vi "CANopen add SDO from EDS.vi"(10 "SDO Parameters in":T4[](array[typedef]) {"Block Data" format="%.0x"}, 11 "Cluster":T2 {"ObjectType" items=[""=10, "NULL"=0, "DOMAIN"=2, "DEFTYPE"=5, "DEFSTRUCT"=6, "VAR"=7, "ARRAY"=8, "RECORD"=9]; "DataType" items=[""=0, "BOOLEAN"=1, "INTEGER8"=2, "INTEGER16"=3, "INTEGER32"=4, "UNSIGNED8"=5, "UNSIGNED16"=6, "UNSIGNED32"=7, "REAL32"=8, "VISIBLE_STRING"=9, "OCTET_STRING"=10, "UNICODE_STRING"=11, "TIME_OF_DAY"=12, "TIME_DIFFERENCE"=13, "DOMAIN"=15, "INTEGER24"=16, "REAL64"=17, "INTEGER40"=18, "INTEGER48"=19, "INTEGER56"=20, "INTEGER64"=21, "UNSIGNED24"=22, "UNSIGNED40"=24, "UNSIGNED48"=25, "UNSIGNED56"=26, "UNSIGNED64"=27]}) -> (2 "SDO Parameters":T4[](array[typedef]) {"Sub-Index (0)" format="%.0x"; "Object Index" format="%.0x"; "Block Data" format="%.0x"})   [LabVIEW 2021, in "CANOpen Addon System Explorer.lvlib"]
uses:
  CANOpen Addon System Explorer.lvlib
  Shared/CANOpen_SDO Settings.ctl
  CANopen SDO EDS data.ctl
  EDS/control/Object Type.ctl
  EDS/control/Data Type.ctl
  CANopen Edit SDO ESD enum.ctl
  Shared/CANOpen Addon Shared.lvlib
panel:
  in  "Translated value float":dbl format="%#_11g"
  in  "Translated value":i64
  out "Default value string":string
  out "Data Type":T1 items=[""=0, "BOOLEAN"=1, "INTEGER8"=2, "INTEGER16"=3, "INTEGER32"=4, "UNSIGNED8"=5, "UNSIGNED16"=6, "UNSIGNED32"=7, "REAL32"=8, "VISIBLE_STRING"=9, "OCTET_STRING"=10, "UNICODE_STRING"=11, "TIME_OF_DAY"=12, "TIME_DIFFERENCE"=13, "DOMAIN"=15, "INTEGER24"=16, "REAL64"=17, "INTEGER40"=18, "INTEGER48"=19, "INTEGER56"=20, "INTEGER64"=21, "UNSIGNED24"=22, "UNSIGNED40"=24, "UNSIGNED48"=25, "UNSIGNED56"=26, "UNSIGNED64"=27]
  in  "Position to import in SDO Parameters array":u16
  in  "Cancel Button":bool
  in  "OK Button":bool
  out "Name":string
  out "Sub-Index (0)":u8 format="%.0x"
  out "Object Index":u16 format="%.0x"
  out "Block Data":u8[](array[numeric]) format="%.0x"
  # "LSB"
  # "MSB"
  # "LSB"
  # "MSB"
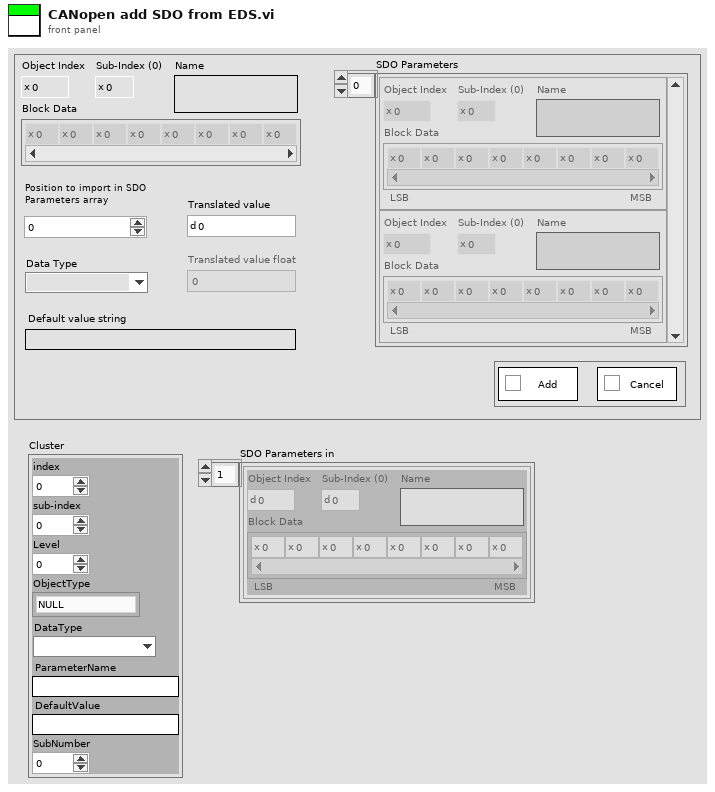
[diagram p1: front panel]
types:
  T1 = typedef "CANOpen Addon System Explorer.lvlib/Data Type.ctl" = u16
  T2 = typedef "CANOpen Addon System Explorer.lvlib/CANopen SDO EDS data.ctl" = cluster{"index":u16, "sub-index":u8, "Level":u8, "ObjectType":T3, "DataType":T1, "ParameterName":string, "DefaultValue":string, "SubNumber":u8}
  T3 = typedef "CANOpen Addon System Explorer.lvlib/Object Type.ctl" = u16
  T4 = typedef "CANOpen Addon Shared.lvlib/CANOpen_SDO Settings.ctl" = cluster{"Object Index":u16, "Sub-Index (0)":u8, "Block Data":u8[], "Name":string}
  T5 = typedef "CANOpen Addon System Explorer.lvlib/CANopen Edit SDO ESD enum.ctl" = enum16{"Init", "Wait", "Insert new item", "Shutdown", "Not supported"}
  T6 = enum8{"Enabled", "Disabled", "Disabled and Grayed Out"}
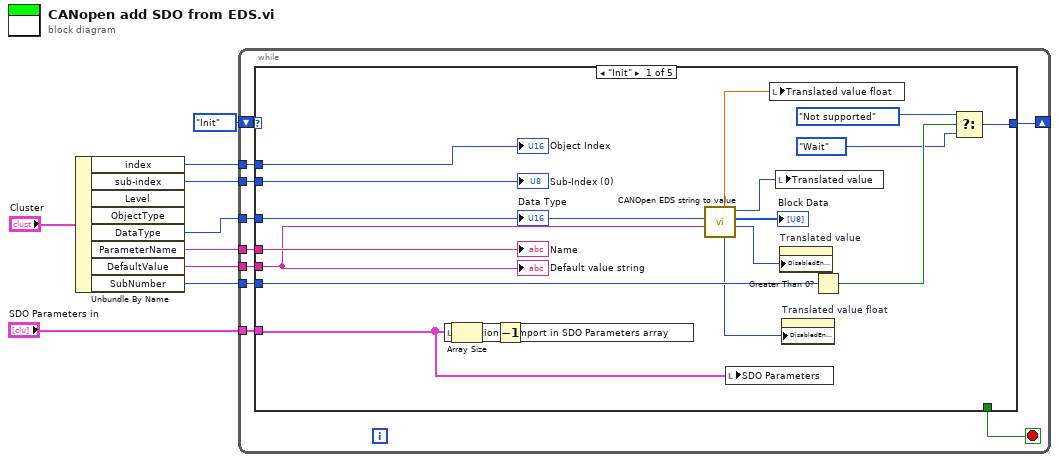
[diagram p0: block diagram]
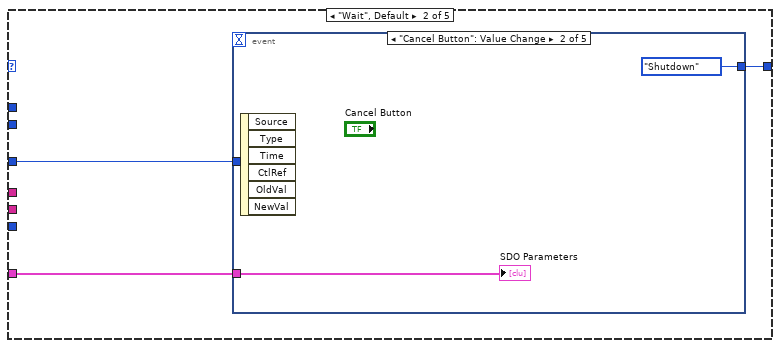
[diagram p2: hidden frame]
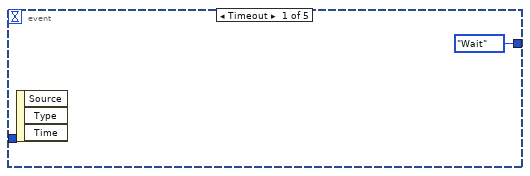
[diagram p3: hidden frame]
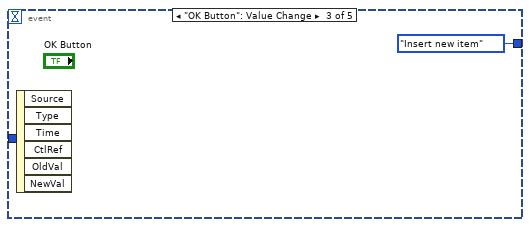
[diagram p4: hidden frame]
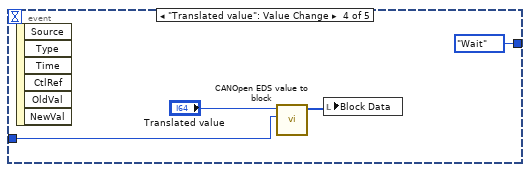
[diagram p5: hidden frame]
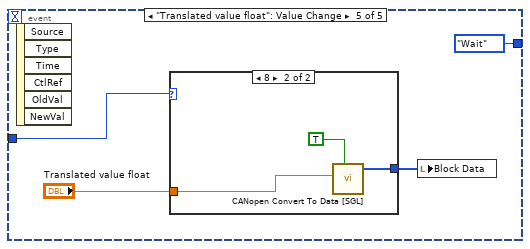
[diagram p6: hidden frame]
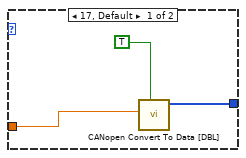
[diagram p7: hidden frame]
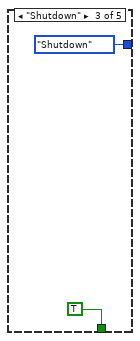
[diagram p8: hidden frame]
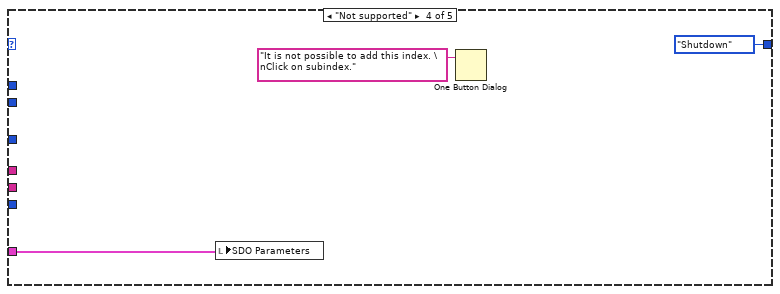
[diagram p9: hidden frame]
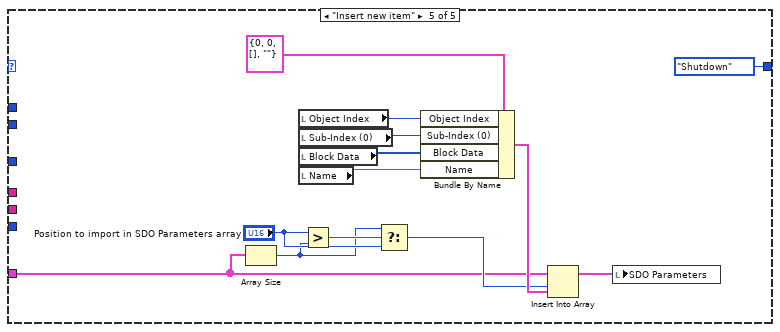
[diagram p10: hidden frame]
diagram:
  n1 = Unbundle By Name("Cluster") -> ("index"=w6:u16, "sub-index"=w5:u8, "DataType"=w2:T1, "ParameterName"=w4:string, "DefaultValue"=w1:string, "SubNumber"=w7:u8)  [unwired: 2 out]
  n2 = while {
    shift-right: [w18] -> _
    shift-left: CANopen_Edit_SDO_ESD_enum."Init" -> [w19]
    tunnel: w7 -> [w16]
    tunnel: w6 -> [w15]
    tunnel: w5 -> [w14]
    tunnel: w4 -> [w13]
    tunnel: "SDO Parameters in" -> [w12]
    tunnel: w2 -> [w11]
    tunnel: w1 -> [w10]
    stop <- w17 stop-if-true
    n3 = case shown="\"Init\"" w19 {
      tunnel: [w34 w39 CANopen_Edit_SDO_ESD_enum."Shutdown" CANopen_Edit_SDO_ESD_enum."Shutdown" CANopen_Edit_SDO_ESD_enum."Shutdown"] -> w18
      tunnel: [_ _ TRUE _ _] -> w17
      tunnel: w16 -> [w36 _ _ _ _]
      tunnel: w15 -> [w31 _ _ _ _]
      tunnel: w14 -> [w30 _ _ _ _]
      tunnel: w13 -> [w29 _ _ _ _]
      tunnel: w12 -> [w20 w38 _ w60 w64]
      tunnel: w11 -> [w25 w37 _ _ _]
      tunnel: w10 -> [w27 _ _ _ _]
      frame "Init" {
        n4 = Array Size(array=w20) -> (size(s)=w28:i32)
        n5 = local write "Position to import in SDO Parameters array"(w28) -> ()
        n6 = Decrement(x=w28) -> ()  [unwired: 1 out]
        n7 = call "CANOpen EDS string to value.vi"("DefaultValue"=w27, "DataType"=w25) -> ("Disabled"=w23:T6, "Block Data"=→"Block Data":u8[], "Translated value"=w26:i64, "Disabled float"=w22:T6, "Translated value float"=w21:dbl)  [unwired: 5 in]
        n8 = local write "SDO Parameters"(w20) -> ()
        n9 = local write "Translated value float"(w21) -> ()
        n10 = local write "Translated value"(w26) -> ()
        n11 = property on="Translated value" class="DigNum (strict)"("DisabledEnum"=w23) -> ()  [unwired: 2 in, 2 out]
        n12 = property on="Translated value float" class="DigNum (strict)"("DisabledEnum"=w22) -> ()  [unwired: 2 in, 2 out]
        n13 = Greater Than 0?(x=w36) -> (x > 0?=w35:bool)
        n14 = Select(t=CANopen_Edit_SDO_ESD_enum."Not supported", s=w35, f=CANopen_Edit_SDO_ESD_enum."Wait") -> (s? t:f=w34:T5)
        "Object Index" <- w31
        "Sub-Index (0)" <- w30
        "Name" <- w29
        "Data Type" <- w25
        "Default value string" <- w27
      }
      frame "Wait", Default {
        n15 = event shown="[1] \"Cancel Button\": Value Change" {
          selector: _ -> [_ _ _ _ _]
          dyn-events: _ -> [_ _ _ _ _]
          timeout: _ -> [_ _ _ _ _]
          tunnel: [CANopen_Edit_SDO_ESD_enum."Wait" CANopen_Edit_SDO_ESD_enum."Shutdown" CANopen_Edit_SDO_ESD_enum."Insert new item" CANopen_Edit_SDO_ESD_enum."Wait" CANopen_Edit_SDO_ESD_enum."Wait"] -> w39
          tunnel: w38 -> [_ w41 _ _ _]
          tunnel: w37 -> [_ _ _ w46 w51]
          event Timeout {
            n16 = event-data() -> ()  [unwired: 1 in, 3 out]
          }
          event "Cancel Button": Value Change {
            n17 = event-data() -> ()  [unwired: 1 in, 6 out]
            "SDO Parameters" <- w41
          }
          event "OK Button": Value Change {
            n18 = event-data() -> ()  [unwired: 1 in, 6 out]
          }
          event "Translated value": Value Change {
            n19 = event-data() -> ()  [unwired: 1 in, 6 out]
            n20 = call "CANOpen EDS value to block.vi"("DataType"=w46, "Translated value"="Translated value") -> ("Block Data"=w47:u8[])  [unwired: 9 in]
            n21 = local write "Block Data"(w47) -> ()
          }
          event "Translated value float": Value Change {
            n22 = event-data() -> ()  [unwired: 1 in, 6 out]
            n23 = case shown="8" w51 {
              tunnel: [w53 w56] -> w49
              tunnel: "Translated value float" -> [w52 w55]
              frame 17, Default {
                n24 = call <vilib>:"CANopen Convert To Data [DBL].vi"("trim"=TRUE, "8-byte double"=w52) -> ("CANopen data out"=w53:u8[])  [unwired: 8 in, 1 out]
              }
              frame 8 {
                n25 = call <vilib>:"CANopen Convert To Data [SGL].vi"("trim"=TRUE, "4-byte single"=w55) -> ("CANopen data out"=w56:u8[])  [unwired: 8 in, 1 out]
              }
            }
            n26 = local write "Block Data"(w49) -> ()
          }
        }
      }
      frame "Shutdown" {
      }
      frame "Not supported" {
        n27 = local write "SDO Parameters"(w60) -> ()
        n28 = One Button Dialog(message="It is not possible to add this index. \nClick on subindex.") -> ()  [unwired: 1 in, 1 out]
      }
      frame "Insert new item" {
        n29 = Array Size(array=w64) -> (size(s)=w63:i32)
        n30 = local read "Object Index"() -> (w71:u16)
        n31 = local read "Sub-Index (0)"() -> (w70:u8)
        n32 = local read "Block Data"() -> (w69:u8[])
        n33 = local read "Name"() -> (w68:string)
        n34 = Greater?(x="Position to import in SDO Parameters array", y=w63) -> (0:w67:bool)
        n35 = Select(t=w63, s=w67, f="Position to import in SDO Parameters array") -> (s? t:f=w65:i32)
        n36 = Bundle By Name(cluster=T4 {"Object Index"=0, "Sub-Index (0)"=0, "Block Data"=[], "Name"=""} ("new element/subarray"), "Object Index"=w71, "Sub-Index (0)"=w70, "Block Data"=w69, "Name"=w68) -> (w72:T4)
        n37 = Insert Into Array(array=w64, index=w65, new element=w72) -> (w74:T4[])
        n38 = local write "SDO Parameters"(w74) -> ()
      }
    }
  }
